vi "generateRandomString.vi"(11 "RandomStringGenerator in":refnum<class "RandomStringGenerator.lvclass">) -> (2 "Random String":string, 3 "RandomStringGenerator out":refnum<class "RandomStringGenerator.lvclass">)   [LabVIEW 2013, in "RandomStringGenerator.lvclass"]
uses:
  RandomStringGenerator.lvclass
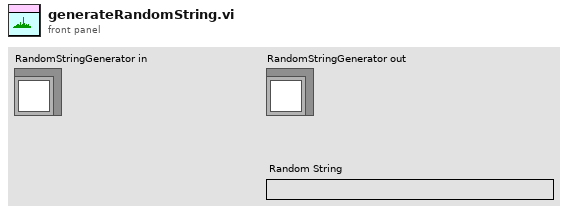
[diagram p1: front panel]
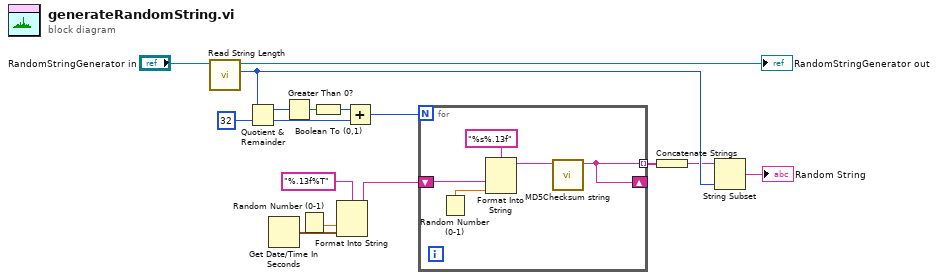
[diagram p0: block diagram]
diagram:
  n1 = call "Read String Length.vi"("RandomStringGenerator in"="RandomStringGenerator in") -> ("String Length"=w8:u32, "RandomStringGenerator out"=→"RandomStringGenerator out":refnum<class "RandomStringGenerator.lvclass">)  [unwired: 9 in]
  n2 = Quotient & Remainder(x=w8, y=u32 32) -> (x-y*floor(x/y)=w13:u32, floor(x/y)=w11:u32)
  n3 = Get Date/Time In Seconds() -> (seconds since 1Jan1904=w2:timestamp)
  n4 = Greater Than 0?(x=w13) -> (x > 0?=w12:bool)
  n5 = Random Number (0-1)() -> (number: 0 to 1=w3:dbl)
  n6 = Boolean To (0,1)(Boolean=w12) -> (0, 1=w10:i16)
  n7 = Format Into String(format string="%.13f%T", w3, w2) -> (resulting string=w4:string)  [unwired: 2 in, 1 out]
  n8 = Add(x=w10, y=w11) -> (x+y=w9:u32)
  n9 = for {
    N: w9 -> [_]
    shift-right: [w21] -> _
    shift-left: w4 -> [w20]
    tunnel: [w21] -> w6 mode=indexing
    n10 = Random Number (0-1)() -> (number: 0 to 1=w17:dbl)
    n11 = Format Into String(format string="%s%.13f", w20, w17) -> (resulting string=w19:string)  [unwired: 2 in, 1 out]
    n12 = call <vilib>:"MD5Checksum string.vi"("Message String"=w19) -> ("MD5 message-digest"=w21:string)  [unwired: 10 in]
  }
  n13 = Concatenate Strings(w6) -> (w5:string)
  n14 = String Subset(string=w5, length (rest)=w8) -> (substring=→"Random String":string)  [unwired: 1 in]
